vi "WritePin.vi"(0 "Simulado in":refnum<class "Simulado.lvclass">, 5 "Port":dbl, 7 "Pin":dbl, 9 "Value":bool, 11 "error in (no error)":errorcluster) -> (4 "Simulado out":refnum<class "Simulado.lvclass">, 15 "error out":errorcluster)   [LabVIEW 2020, in "Simulado.lvclass"]
uses:
  Simulado.lvclass
  Abstract/Serial Device/Serial Device.lvclass
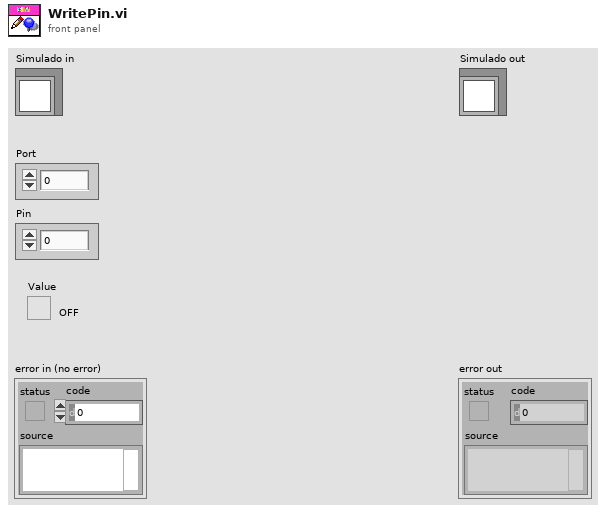
[diagram p1: front panel]
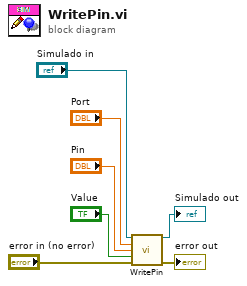
[diagram p0: block diagram]
diagram:
  n1 = call-parent "WritePin.vi"("Serial Device in"="Simulado in", "Port"="Port", "Pin"="Pin", "Value"="Value", "error in (no error)"="error in (no error)") -> ("Serial Device out"=→"Simulado out":refnum<class "Simulado.lvclass">, "error out"=→"error out":errorcluster)  [unwired: 9 in]
